vi "Write Digital Out State.vi"(8 "error in":errorcluster, 9 "Selection":i32, 10 "Value":bool, 11 "PLC in":refnum<class "PLC.lvclass">) -> (0 "error out":errorcluster, 3 "PLC out":refnum<class "PLC.lvclass">)   [LabVIEW 2018, in "PLC.lvlib" / "PLC.lvclass"]
uses:
  PLC.lvclass
  Custom Controls/Selector.ctl
  PLC.lvclass/PLC.ctl
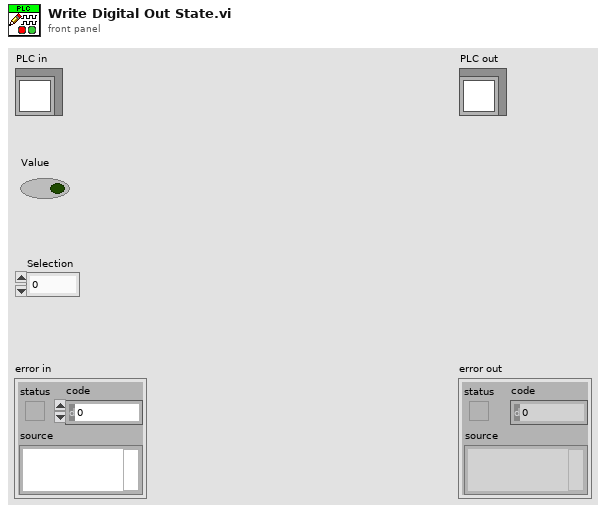
[diagram p1: front panel]
types:
  T1 = typedef "PLC.lvlib/PLC.lvclass/Selector.ctl" = enum16{"Digital", "Analog"}
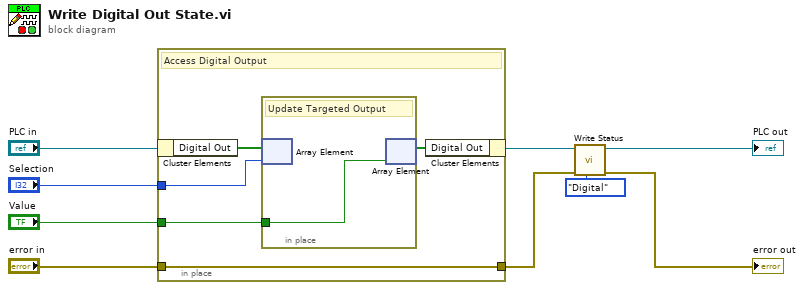
[diagram p0: block diagram]
diagram:
  n1 = in-place {
    in-place-border: "Selection" -> [w14]
    in-place-border: "Value" -> [w13]
    in-place-border: "error in" -> [w10]
    in-place-border: [w10] -> w1
    # "Access Digital Output"
    n2 = in-place-cluster #1("PLC in") -> ("Digital Out"=w12:bool[])
    n3 = in-place {
      in-place-border: w13 -> [w15]
      # "Update Targeted Output"
      n4 = in-place-array #2(w12, w14) -> ()  [unwired: 1 out]
      n5 = in-place-array #2(w15) -> (w11:bool[])  [unwired: 1 out]
    }
    n6 = in-place-cluster #1("Digital Out"=w11) -> (w3:refnum<class "PLC.lvclass">)
  }
  n7 = call-dynamic "Write Status.vi"("Selector"=Selector."Digital", "error in"=w1, "PLC in"=w3) -> ("error out"=→"error out":errorcluster, "PLC out"=→"PLC out":refnum<class "PLC.lvclass">)  [unwired: 7 in]
